vi "Temperature Limit.vi"() -> ()   [LabVIEW 2015]
doc: "This VI simulates the acquisition of temperature, graphs the temperature, and notifies the user if the temperature is over the limit."
panel:
  in  "Start":bool
  in  "Delta t (ms)":i32(slide)=400 scale=50.0..500.0
  in  "Stop":bool
  in  "High Limit":dbl=28.0 format="%.2f"
  out "Temperature":cluster{"Temperature":dbl, "High Limit":dbl}(graph)={"Temperature"=85.88749999999999, "High Limit"=80.0}
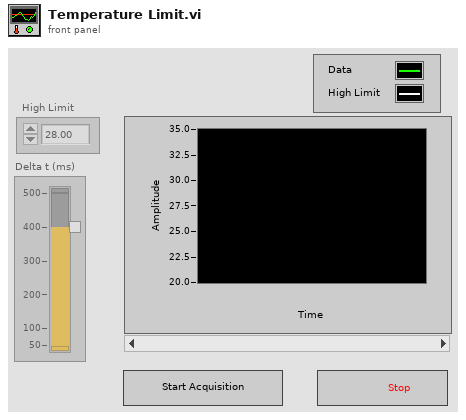
[diagram p1: front panel]
types:
  T1 = enum16{"Always On", "Always Off", "Off While Running"}
  T2 = enum8{"Enabled", "Disabled", "Disabled and Grayed Out"}
  T3 = cluster{"Temperature Value":dbl, "High Limit":dbl}
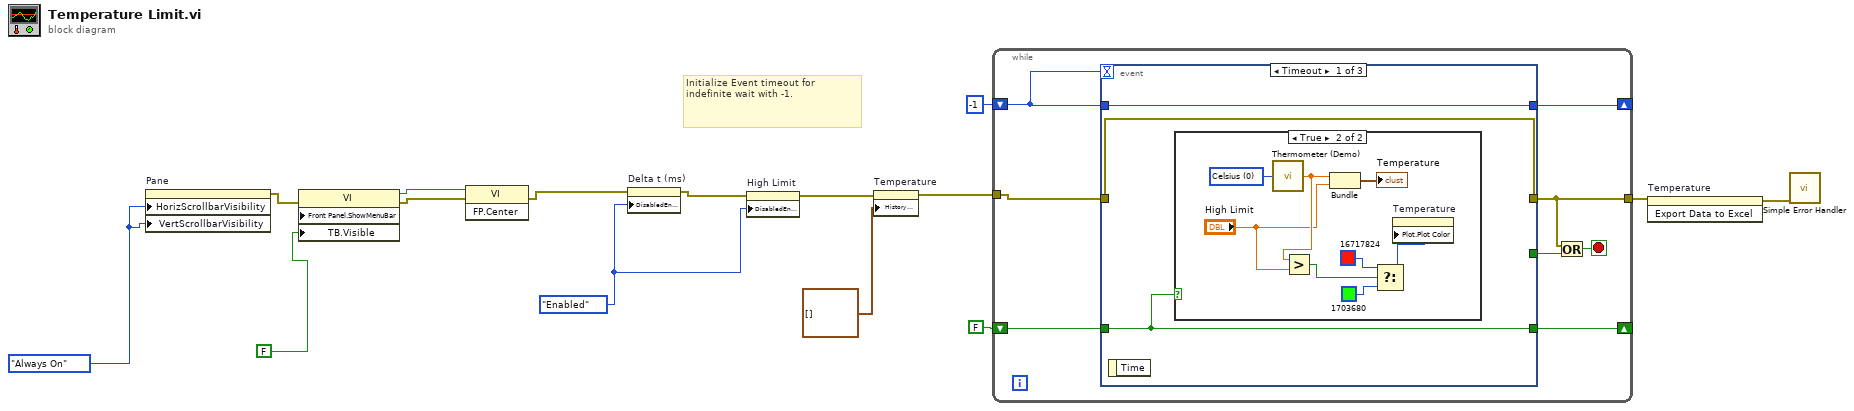
[diagram p0: block diagram]
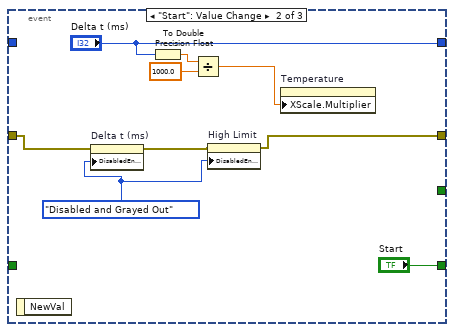
[diagram p3: hidden frame]
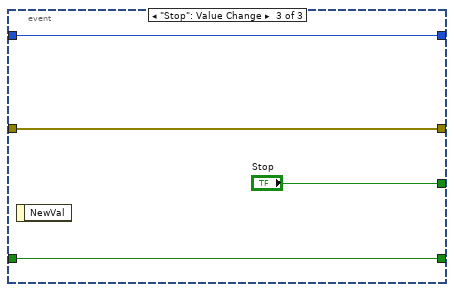
[diagram p4: hidden frame]
diagram:
  w7 = FALSE ("Front Panel Window:Show Menu Bar")
  w8 = T1."Always On" ("Horizontal Scrollbar Visibility")
  w12 = T2."Enabled" ("Disabled")
  # "Initialize Event timeout for indefinite wait with -1."
  n1 = property on="Pane" class="Pane"("HorizScrollbarVisibility"=w8, "VertScrollbarVisibility"=w8) -> (error out=w6:errorcluster)  [unwired: 2 in, 1 out]
  n2 = property class="VI"(error in=w6, "Front Panel.ShowMenuBar"=w7, "TB.Visible"=w7) -> (reference out=w3:refnum<vi>, error out=w5:errorcluster)  [unwired: 1 in]
  n3 = invoke class="VI" method="FP.Center"(reference=w3, error in=w5) -> (error out=w4:errorcluster)  [unwired: 1 in, 2 out]
  n4 = property on="Delta t (ms)" class="Slide (strict)"(error in=w4, "DisabledEnum"=w12) -> (error out=w13:errorcluster)  [unwired: 1 in, 1 out]
  n5 = property on="High Limit" class="DigNum (strict)"(error in=w13, "DisabledEnum"=w12) -> (error out=w11:errorcluster)  [unwired: 1 in, 1 out]
  n6 = property on="Temperature" class="WFChart (strict)"(error in=w11, "History Data"=cluster{"Temperature":dbl, "High Limit":dbl}[] []) -> (error out=w10:errorcluster)  [unwired: 1 in, 1 out]
  n7 = while {
    tunnel: [w22] -> w2
    shift-right: [w20] -> _
    shift-left: FALSE ("Start") -> [w19]
    shift-right: [w18] -> _
    shift-left: -1 ("Delta t (ms)") -> [w17]
    tunnel: w10 -> [w16]
    stop <- w23 stop-if-true
    n8 = event shown="[0] Timeout" {
      selector: _ -> [_ _ _]
      dyn-events: _ -> [_ _ _]
      timeout: w17 -> [_ _ _]
      tunnel: [_ _ "Stop"] -> w21
      tunnel: w16 -> [w26 w42 w46]
      tunnel: [w26 w40 w46] -> w22
      tunnel: [w24 "Start" w45] -> w20
      tunnel: w19 -> [w24 _ w45]
      tunnel: [w25 "Delta t (ms)" w44] -> w18
      tunnel: w17 -> [w25 _ w44]
      event Timeout {
        n9 = event-data() -> ()  [unwired: 1 in, 1 out]
        n10 = case shown="True" w24 {
          frame False {
          }
          frame True {
            w33 = u16 0 items=["Celsius", "Fahrenheit"] ("Units (0: Celsius)")
            n11 = call "Thermometer (Demo).vi"("Units (0: Celsius)"=w33) -> ("Temperature Value"=w32:dbl)
            n12 = Greater?(x=w32, y="High Limit") -> (0:w30:bool)
            n13 = Bundle("Temperature Value"=w32, "High Limit"="High Limit") -> (→"Temperature":T3)  [unwired: 1 in]
            n14 = Select(t=u32 16717824, s=w30, f=u32 1703680) -> (s? t:f=w29:u32)
            n15 = property on="Temperature" class="WFChart (strict)"("Plot.Plot Color"=w29) -> ()  [unwired: 2 in, 2 out]
          }
        }
      }
      event "Start": Value Change {
        w39 = T2."Disabled and Grayed Out" ("Disabled")
        n16 = event-data() -> ()  [unwired: 1 in, 1 out]
        n17 = property on="Delta t (ms)" class="Slide (strict)"(error in=w42, "DisabledEnum"=w39) -> (error out=w41:errorcluster)  [unwired: 1 in, 1 out]
        n18 = To Double Precision Float(number="Delta t (ms)") -> (double precision float=w37:dbl)
        n19 = Divide(x=w37, y=1000.0) -> (x/y=w35:dbl)
        n20 = property on="High Limit" class="DigNum (strict)"(error in=w41, "DisabledEnum"=w39) -> (error out=w40:errorcluster)  [unwired: 1 in, 1 out]
        n21 = property on="Temperature" class="WFChart (strict)"("XScale.Multiplier"=w35) -> ()  [unwired: 2 in, 2 out]
      }
      event "Stop": Value Change {
        n22 = event-data() -> ()  [unwired: 1 in, 1 out]
      }
    }
    n23 = Or(x=w22, y=w21) -> (x .or. y?=w23:bool)
  }
  n24 = invoke on="Temperature" class="WFChart (strict)" method="Export Data to Excel"(error in=w2) -> (error out=w1:errorcluster)  [unwired: 2 in, 2 out]
  n25 = call <vilib>:"Simple Error Handler.vi"("error in (no error)"=w1) -> ()  [unwired: 4 in, 5 out]
